vi "Post ECL Entry.vi"(4 "password":string, 6 "username":string, 7 "Category":T1(ring), 8 "error in (no error)":errorcluster, 9 "Image Attachements":path[](array[path]), 10 "File Attachements":path[](array[path]), 11 "Entry Text":string) -> (0 "error out":errorcluster, 2 "Entry ID":i32)   [LabVIEW 2013]
uses:
  <vilib>/httpClient/POSTBuffer.vi
  <vilib>/httpClient/LabVIEWHTTPClient.lvlib
panel:
  out "Entry XML":string
  out "body":string
  out "headers":string
  out "ECL Post URL":string
  in  "ECL Base Path":string="ECL/mta"
  in  "ECL Port":u16=8443
  in  "ECL Server":string="dbweb4.fnal.gov"
  # "Post ECL Entry\nupdated 10 Feb 2015\nby P. Lane"
  # "Posts an entry to the MTA ECL"
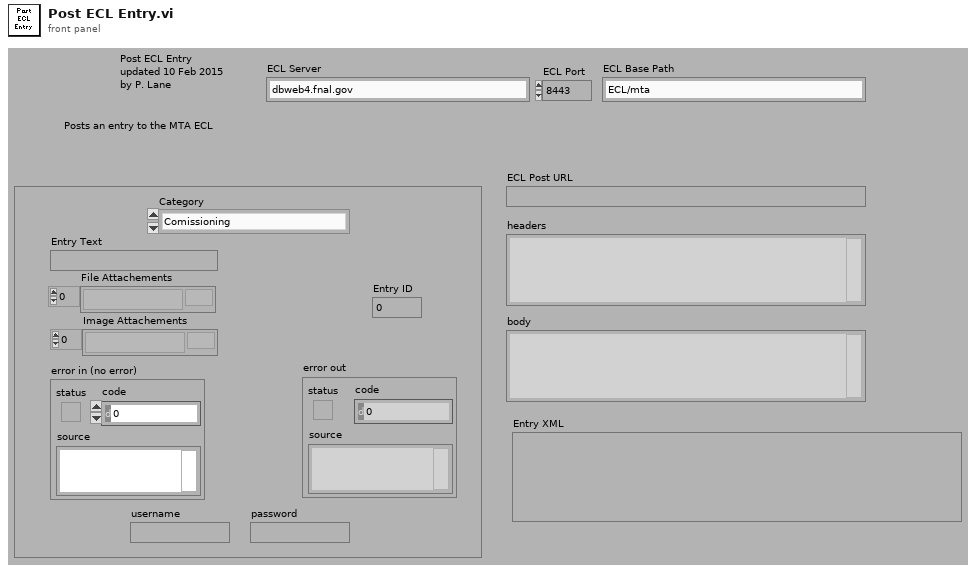
[diagram p1: front panel]
types:
  T1 = enum16{"Comissioning", "Comissioning/Detector", "Operations", "Operations/Absorber", "Operations/Beamline", "Operations/Controls", "Operations/Cryo", "Operations/DAQ", "Operations/Detectors", "Operations/Electrical", "Operations/Magnets", "Operations/Mechanical", "Operations/RF", "Operations/RF/201MHz", "Operations/RF/805MHz", "Operations/RF/PressurizedRF", "Operations/Safety", "Projects", "Projects/Logbook_Comments", "Projects/MTA_Operations", "Projects/MTA_Operations/Sandbox", "Sandbox", "Sandbox/Log", "Studies", "Studies/2010", "Studies/2010/2011_HPRF_test"}
  T2 = typedef "LabVIEWHTTPClient.lvlib/ClientHandle.ctl" = refnum<k1>
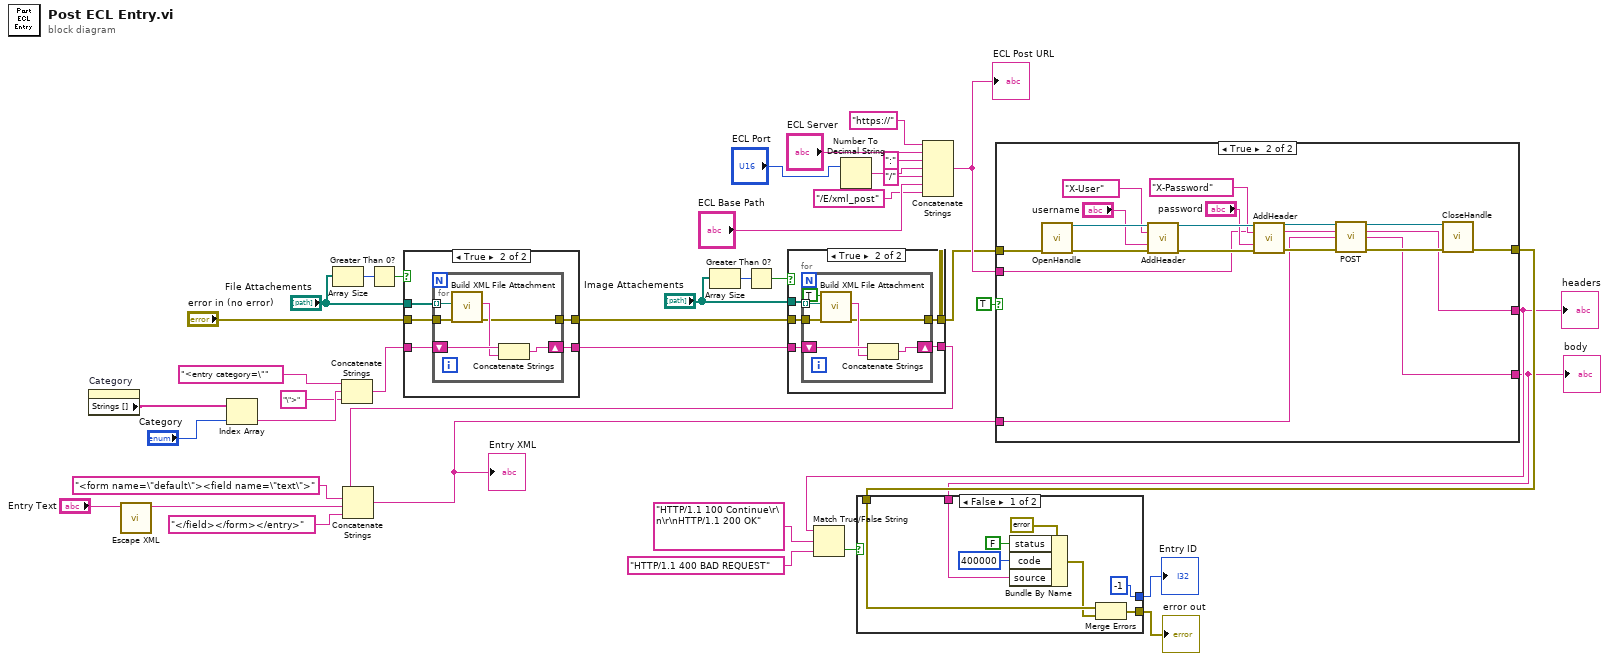
[diagram p0: block diagram]
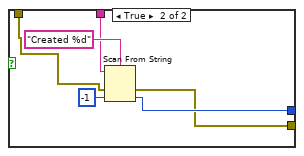
[diagram p2: hidden frame]
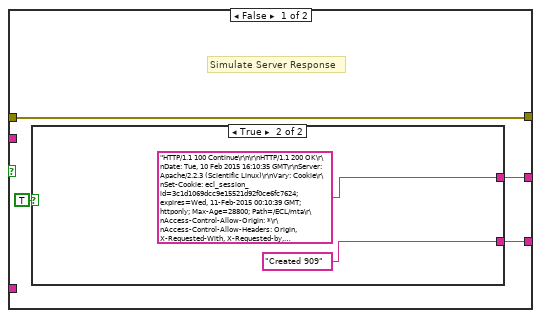
[diagram p5: hidden frame]
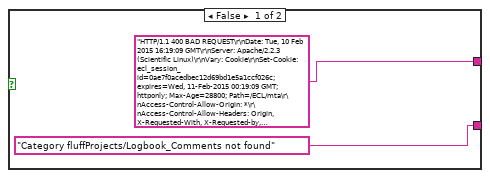
[diagram p6: hidden frame]
diagram:
  n1 = property on="Category" class="Enum (strict)"() -> ("Strings []"=w27:string[])  [unwired: 2 in, 2 out]
  n2 = call <vilib>:"Escape XML.vi"("XML String In"="Entry Text") -> ("XML String Out"=w1:string)  [unwired: 9 in, 1 out]
  n3 = Index Array(array=w27, index="Category") -> (element=w29:string)
  n4 = Array Size(array="File Attachements") -> (size(s)=w16:i32)
  n5 = Concatenate Strings("<entry category=\"", w29, "\">") -> (w24:string)
  n6 = Greater Than 0?(x=w16) -> (x > 0?=w17:bool)
  n7 = case shown="True" w17 {
    tunnel: "File Attachements" -> [_ w47]
    tunnel: "error in (no error)" -> [w41 w46]
    tunnel: w24 -> [w42 w45]
    tunnel: [w41 w44] -> w23
    tunnel: [w42 w43] -> w22
    frame False {
    }
    frame True {
      n8 = for {
        tunnel: w47 -> [w53] mode=indexing
        tunnel: w46 -> [w52]
        shift-right: [w49] -> w43
        shift-left: w45 -> [w51]
        tunnel: [w48] -> w44
        n9 = call "Build XML File Attachment.vi"("error in"=w52, "file"=w53) -> ("error out"=w48:errorcluster, "string out (XML Attachment))"=w50:string)  [unwired: 8 in]
        n10 = Concatenate Strings(w51, w50) -> (w49:string)
      }
    }
  }
  n11 = Array Size(array="Image Attachements") -> (size(s)=w14:i32)
  n12 = Greater Than 0?(x=w14) -> (x > 0?=w12:bool)
  n13 = case shown="True" w12 {
    tunnel: w23 -> [w54 w60]
    tunnel: w22 -> [w55 w59]
    tunnel: [w55 w56] -> w21
    tunnel: [w54 w58] -> w18
    tunnel: "Image Attachements" -> [_ w57]
    frame False {
    }
    frame True {
      n14 = for {
        tunnel: w57 -> [w67] mode=indexing
        tunnel: w60 -> [w66]
        shift-right: [w62] -> w56
        shift-left: w59 -> [w65]
        tunnel: [w63] -> w58
        n15 = call "Build XML File Attachment.vi"("error in"=w66, "file"=w67, "Image (false)"=TRUE) -> ("error out"=w63:errorcluster, "string out (XML Attachment))"=w64:string)  [unwired: 7 in]
        n16 = Concatenate Strings(w65, w64) -> (w62:string)
      }
    }
  }
  n17 = Concatenate Strings(w21, "<form name=\"default\"><field name=\"text\">" ("string"), w1, "</field></form></entry>" ("string")) -> (w3:string)
  "Entry XML" <- w3
  n18 = Number To Decimal String(number="ECL Port") -> (decimal integer string=w36:string)  [unwired: 1 in]
  n19 = Concatenate Strings("https://" ("string"), "ECL Server", ":" ("string"), w36, "/" ("string"), "ECL Base Path", "/E/xml_post" ("string")) -> (w33:string)
  "ECL Post URL" <- w33
  n20 = case shown="True" TRUE {
    tunnel: w33 -> [_ w81]
    tunnel: w18 -> [w71 w80]
    tunnel: [w71 w79] -> w8
    tunnel: w3 -> [_ w78]
    tunnel: [w70 w77] -> w6
    tunnel: [w69 w76] -> w5
    frame False {
      # "Simulate Server Response"
      n21 = case shown="True" TRUE {
        tunnel: ["HTTP/1.1 400 BAD REQUEST\r\nDate: Tue, 10 Feb 2015 16:19:09 GMT\r\nServer: Apache/2.2.3 (Scientific Linux)\r\nVary: Cookie\r\nSet-Cookie: ecl_session_id=0ae7f0acedbec12d69bd1e5a1ccf026c; expires=Wed, 11-Feb-2015 00:19:09 GMT; httponly; Max-Age=28800; Path=/ECL/mta\r\nAccess-Control-Allow-Origin: *\r\nAccess-Control-Allow-Headers: Origin, X-Requested-With, X-Requested-by, Content-Type, Accept, X-Request\r\nContent-Length: 49\r\nConnection: close\r\nContent-Type: text/html; charset=utf-8\r\n\r\n" ("headers") "HTTP/1.1 100 Continue\r\n\r\nHTTP/1.1 200 OK\r\nDate: Tue, 10 Feb 2015 16:10:35 GMT\r\nServer: Apache/2.2.3 (Scientific Linux)\r\nVary: Cookie\r\nSet-Cookie: ecl_session_id=3c1d1069dcc9e15521d92f0ce6fc7624; expires=Wed, 11-Feb-2015 00:10:39 GMT; httponly; Max-Age=28800; Path=/ECL/mta\r\nAccess-Control-Allow-Origin: *\r\nAccess-Control-Allow-Headers: Origin, X-Requested-With, X-Requested-by, Content-Type, Accept, X-Request\r\nContent-Length: 12\r\nConnection: close\r\nContent-Type: text/html; charset=utf-8\r\n\r\n" ("headers")] -> w70
        tunnel: ["Category fluffProjects/Logbook_Comments not found" ("body") "Created 909" ("body")] -> w69
        frame False {
        }
        frame True {
        }
      }
    }
    frame True {
      n22 = call <vilib>:"OpenHandle.vi"("error in (no error)"=w80) -> ("client handle out"=w93:T2, "error out"=w90:errorcluster)  [unwired: 13 in]
      n23 = call <vilib>:"AddHeader.vi"("client handle"=w93, "header"="X-User", "value"="username", "error in (no error)"=w90) -> ("client handle out"=w89:T2, "error out"=w88:errorcluster)  [unwired: 10 in]
      n24 = call <vilib>:"AddHeader.vi"("client handle"=w89, "header"="X-Password", "value"="password", "error in (no error)"=w88) -> ("client handle out"=w85:T2, "error out"=w84:errorcluster)  [unwired: 10 in]
      n25 = call-poly <vilib>:"POST.vi"("client handle"=w85, "url"=w81, "buffer"=w78, "error in (no error)"=w84) -> ("client handle out"=w82:T2, "headers"=w77:string, "body"=w76:string, "error out"=w83:errorcluster)  [unwired: 8 in]
      n26 = call <vilib>:"CloseHandle.vi"("client handle"=w82, "error in (no error)"=w83) -> ("error out"=w79:errorcluster)  [unwired: 13 in]
    }
  }
  "headers" <- w6
  "body" <- w5
  n27 = Match True/False String(2:"HTTP/1.1 400 BAD REQUEST" ("headers"), 3:"HTTP/1.1 100 Continue\r\n\r\nHTTP/1.1 200 OK" ("headers"), 4:w6) -> (0:w9:bool)  [unwired: 1 out]
  n28 = case shown="False" w9 {
    tunnel: w5 -> [w96 w106]
    tunnel: w8 -> [w99 w104]
    tunnel: [-1 ("default value 1") w103] -> w7
    tunnel: [w100 w102] -> w4
    frame False {
      n29 = Bundle By Name(cluster=errorcluster {"status"=FALSE, "code"=0, "source"=""} ("error constant"), "status"=FALSE, "code"=400000, "source"=w96) -> (w94:errorcluster)
      n30 = Merge Errors(w99, w94) -> (w100:errorcluster)
    }
    frame True {
      n31 = Scan From String(format string="Created %d", input string=w106, error in=w104, default 1=-1 ("default value 1")) -> (error out=w102:errorcluster, output 1=w103:i32)  [unwired: 1 in, 2 out]
    }
  }
  "error out" <- w4
  "Entry ID" <- w7
